vi "1111_#ROTATO.vi"(8 "Refnum in":refnum<k33>, 11 "Degrees":dbl=90.0) -> (0 "rt fifo out":refnum<k33>)   [LabVIEW 2014]
uses:
  TeleopCmd.ctl
  CmdFlag.ctl
panel:
  in  "Limit":dbl=0.35
  out "error out":errorcluster
  in  "Thresh":dbl=0.5
  in  "Offset":dbl=0.15
  in  "Kp":dbl=0.03
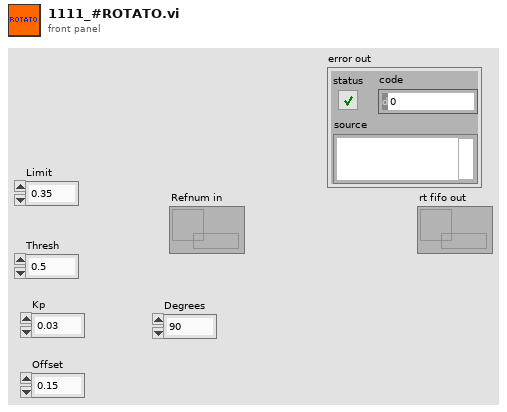
[diagram p1: front panel]
types:
  T1 = typedef "TeleopCmd.ctl" = cluster{"CmdFlag":T2, "throttle":dbl, "turn":dbl, "Override":bool, "Strafe":dbl, "MotorPwrMax":u8, "Time":u32, "ultrasonic override":bool}
  T2 = typedef "CmdFlag.ctl" = enum16{"noop", "logflag", "suspend", "resume"}
  T3 = typedef "navX-MXP IMU.lvlib/navX YPRH Data.ctl" = cluster{"Yaw":dbl, "Pitch":dbl, "Roll":dbl, "Heading":dbl}
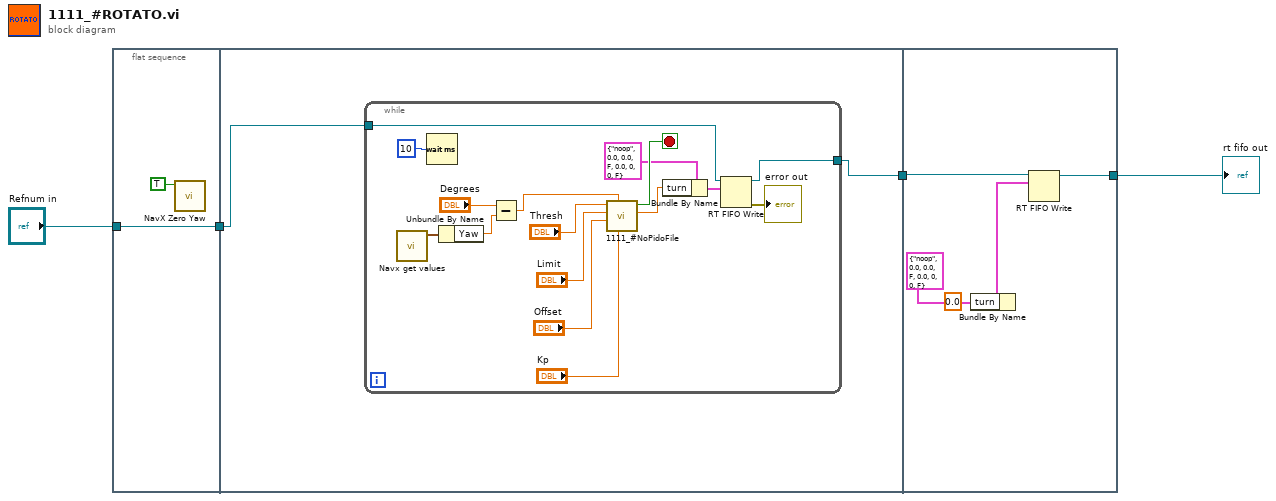
[diagram p0: block diagram]
diagram:
  n1 = flat-sequence {
    tunnel: [w5] -> w4
    tunnel: "Refnum in" -> [w5]
    tunnel: w4 -> [w7]
    tunnel: [w8] -> w1
    tunnel: [w29] -> w2
    tunnel: w1 -> [w28]
    frame #0 {
      n2 = call "NavX Zero Yaw.vi"("Reset NavX Yaw"=TRUE) -> ()  [unwired: 11 in]
    }
    frame #1 {
      n3 = while {
        tunnel: [w22] -> w8
        tunnel: w7 -> [w21]
        stop <- w23 stop-if-true
        n4 = call "Navx get values.vi"() -> ("YPRH"=w24:T3)  [unwired: 11 in]
        n5 = Wait (ms)(milliseconds to wait=u32 10) -> ()  [unwired: 1 out]
        n6 = Unbundle By Name(w24) -> ("Yaw"=w13:dbl)
        n7 = Subtract(x="Degrees", y=w13) -> (x-y=w12:dbl)
        n8 = call "1111_#NoPidoFile.vi"("Kp"="Kp", "error"=w12, "Offset"="Offset", "Limit in"="Limit", "Thresh"="Thresh") -> ("Limit out"=w10:dbl, "Boolean"=w23:bool)  [unwired: 5 in]
        n9 = Bundle By Name(cluster=T1 {"CmdFlag"=enum."noop", "throttle"=0.0, "turn"=0.0, "Override"=FALSE, "Strafe"=0.0, "MotorPwrMax"=0, "Time"=0, "ultrasonic override"=FALSE} ("Cluster"), "turn"=w10) -> (w18:T1)
        n10 = RT FIFO Write(0:w21, 1:w18) -> (8:w22:refnum<k33>, 11:→"error out":errorcluster)  [unwired: 3 in, 2 out]
      }
    }
    frame #2 {
      n11 = Bundle By Name(cluster=T1 {"CmdFlag"=enum."noop", "throttle"=0.0, "turn"=0.0, "Override"=FALSE, "Strafe"=0.0, "MotorPwrMax"=0, "Time"=0, "ultrasonic override"=FALSE} ("Cluster"), "turn"=0.0) -> (w26:T1)
      n12 = RT FIFO Write(0:w28, 1:w26) -> (8:w29:refnum<k33>)  [unwired: 3 in, 3 out]
    }
  }
  "rt fifo out" <- w2
